vi "getImageCamera.vi"(4 "Mostrar?":bool, 5 "Streeam?":bool, 6 "Image Device IN":cluster{"Image":T2, "errorImage":errorcluster}, 7 "Camera Device  IN":T1) -> (1 "Contraste OUT":dbl, 2 "Image Device OUT":cluster{"Image":T2, "errorImage":errorcluster}, 3 "Camera Device OUT":T1)   [LabVIEW 2010]
uses:
  <vilib>/vision/NI_Vision_Development_Module.lvlib
  <vilib>/vision/Image Controls.llb/IMAQ Image.ctl
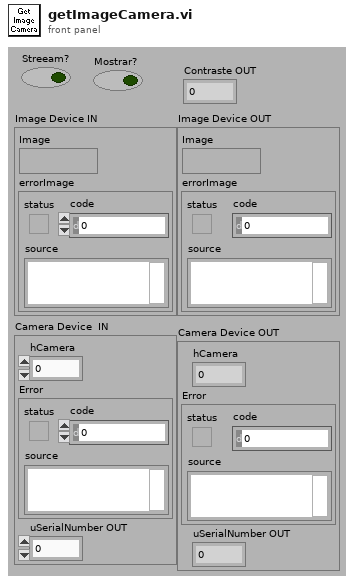
[diagram p1: front panel]
types:
  T1 = cluster{"hCamera":u32, "Error":errorcluster, "uSerialNumber OUT":u32}
  T2 = typedef "IMAQ Image.ctl" = refnum<image>
  T3 = cluster{"hCamera":u32, "Error":errorcluster, "uSerialNumber":u32}
  T4 = cluster{"Red (or Hue) value":u8, "Green (or Sat) value":u8, "Blue (or Light or Val) value":u8}[]
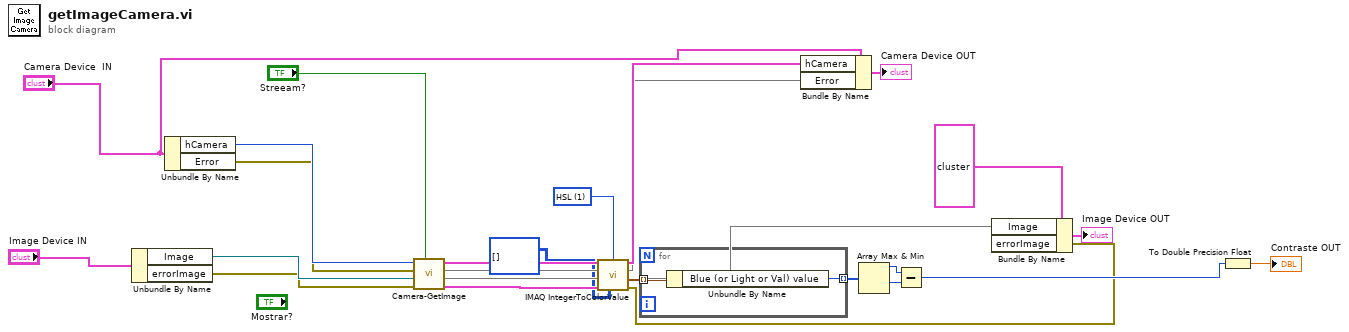
[diagram p0: block diagram]
diagram:
  w19 = u16 1 items=["RGB", "HSL", "HSV", "HSI"] ("Color Mode")
  n1 = Unbundle By Name("Image Device IN") -> ("Image"=w12:T2, "errorImage"=w11:errorcluster)
  n2 = Unbundle By Name("Camera Device  IN") -> ("hCamera"=w15:u32, "Error"=w14:errorcluster)
  n3 = call "Camera-GetImage.vi"("Streeam"="Streeam?", "Image Device IN"=w11, 6:w12, 7:w14, "Camera Device IN"=w15) -> ("Image Device OUT"=w3:cluster{"Image":T2, "errorImage":errorcluster}, 1:w2, 2:w9, "Camera Device OUT"=w10:T3)
  n4 = call "IMAQ IntegerToColorValue"("error in (no error)"=w3, "2D U32 array"=u32[][] [], "Color Mode"=w19) -> ("1D Color value array"=w20:T4, "error out"=w7:errorcluster)  [unwired: 2 in, 2 out]
  n5 = for {
    tunnel: w20 -> [w25] mode=indexing
    tunnel: [w24] -> w21 mode=indexing
    n6 = Unbundle By Name(w25) -> ("Blue (or Light or Val) value"=w24:u8)
  }
  n7 = Bundle By Name(cluster="Camera Device  IN", "hCamera"=w10, "Error"=w9) -> (→"Camera Device OUT":T1)
  n8 = Array Max & Min(array=w21) -> (max value=w22:u8, min value=w23:u8)  [unwired: 2 out]
  n9 = Subtract(x=w22, y=w23) -> (x-y=w16:u8)
  n10 = Bundle By Name(cluster=cluster{"Image":T2, "errorImage":errorcluster} {"Image"=refnum, "errorImage"={"status"=FALSE, "code"=0, "source"=""}} ("Image Device"), "Image"=w2, "errorImage"=w7) -> (→"Image Device OUT":cluster{"Image":T2, "errorImage":errorcluster})
  n11 = To Double Precision Float(number=w16) -> (double precision float=→"Contraste OUT":dbl)
